vi "Set Root.vi"(8 "error in (no error)":errorcluster, 9 "Root Path":path, 10 "Root Name":string, 11 "File Tree In":refnum<class "File Tree.lvclass">) -> (0 "error out":errorcluster, 3 "File Tree Out":refnum<class "File Tree.lvclass">)   [LabVIEW 2020, in "Tree Helpers.lvlib" / "File Tree.lvclass"]
uses:
  File Tree.lvclass
  File Tree.lvclass/File Tree.ctl
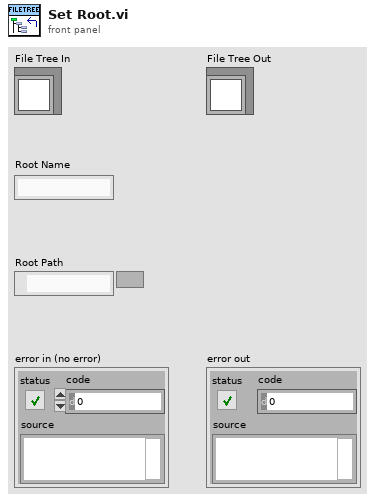
[diagram p1: front panel]
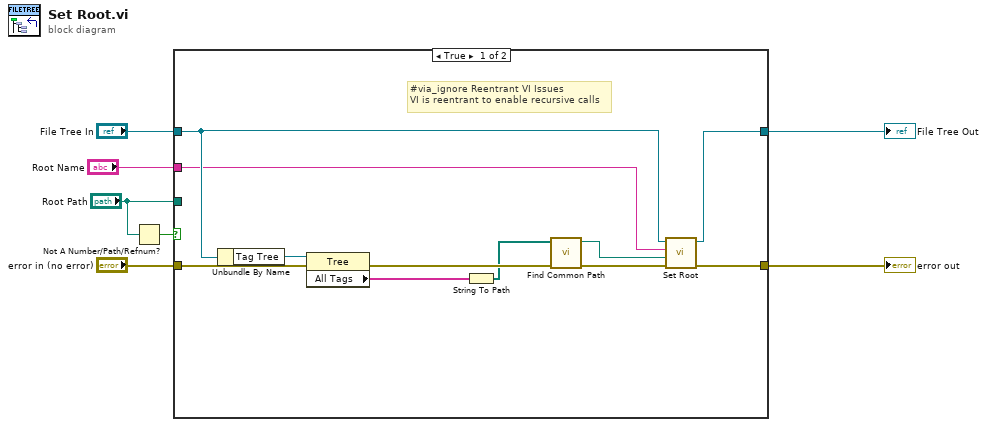
[diagram p0: block diagram]
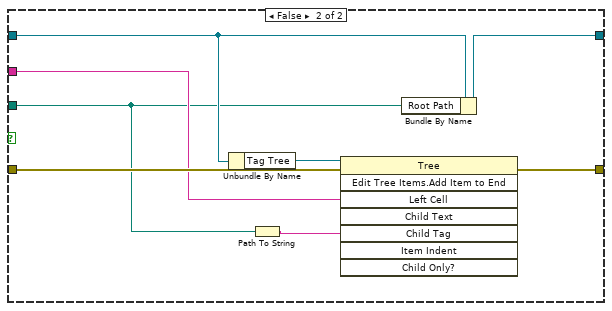
[diagram p2: hidden frame]
diagram:
  n1 = Not A Number/Path/Refnum?(number/path/refnum="Root Path") -> (NaN/Path/Refnum?=w2:bool)
  n2 = case shown="True" w2 {
    tunnel: [w15 w26] -> w7
    tunnel: "File Tree In" -> [w16 w25]
    tunnel: [w14 w24] -> w5
    tunnel: "error in (no error)" -> [w18 w23]
    tunnel: "Root Name" -> [w13 w21]
    tunnel: "Root Path" -> [_ w19]
    frame True {
      # "#via_ignore Reentrant VI Issues\nVI is reentrant to enable recursive calls"
      n3 = Unbundle By Name(w16) -> ("Tag Tree"=w17:refnum<vi>)
      n4 = property on="Property Node" class="Tree"(reference=w17, error in=w18) -> (error out=w12:errorcluster, "All Tags"=w11:string[])  [unwired: 1 out]
      n5 = String To Path(string=w11) -> (path=w10:path[])
      n6 = call "Find Common Path.vi"("error in (no error)"=w12, "File Paths"=w10) -> ("error out"=w8:errorcluster, "Common Path"=w9:path)  [unwired: 8 in]
      n7 = call "Set Root.vi"("error in (no error)"=w8, "Root Path"=w9, "Root Name"=w13, "File Tree In"=w16) -> ("error out"=w14:errorcluster, "File Tree Out"=w15:refnum<class "File Tree.lvclass">)  [unwired: 6 in]
    }
    frame False {
      n8 = Unbundle By Name(w25) -> ("Tag Tree"=w22:refnum<vi>)
      n9 = Path To String(path=w19) -> (string=w20:string)
      n10 = invoke on="Invoke Node" class="Tree" method="Edit Tree Items.Add Item to End"(reference=w22, error in=w23, "Left Cell"=w21, "Child Tag"=w20) -> (error out=w24:errorcluster)  [unwired: 4 in, 7 out]
      n11 = Bundle By Name(cluster=w25, "Root Path"=w19) -> (w26:refnum<class "File Tree.lvclass">)
    }
  }
  "File Tree Out" <- w7
  "error out" <- w5
